vi "Create Tree.vi"(8 "Error In":errorcluster, 10 "Eulogy Bookmarks":T1[](array[typedef]), 11 "TreeControl In":refnum<vi>) -> (0 "Error Out":errorcluster, 3 "TreeControl Out":refnum<vi>)   [LabVIEW 2017, in "Bookmark Manager.lvlib"]
uses:
  Bookmark Manager.lvlib
  Controls/VI Bookmark.ctl
  Controls/VI Information.ctl
  Controls/Application Information.ctl
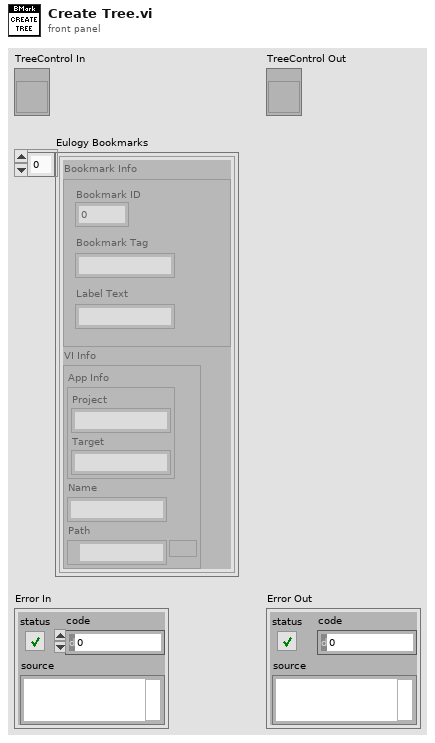
[diagram p1: front panel]
types:
  T1 = typedef "Bookmark Manager.lvlib/VI Bookmark.ctl" = cluster{"Bookmark Info":cluster{"Bookmark ID":u32, "Bookmark Tag":string, "Label Text":string}, "VI Info":T2}
  T2 = typedef "Bookmark Manager.lvlib/VI Information.ctl" = cluster{"App Info":T3, "Name":string, "Path":path}
  T3 = typedef "Bookmark Manager.lvlib/Application Information.ctl" = cluster{"Project":string, "Target":string}
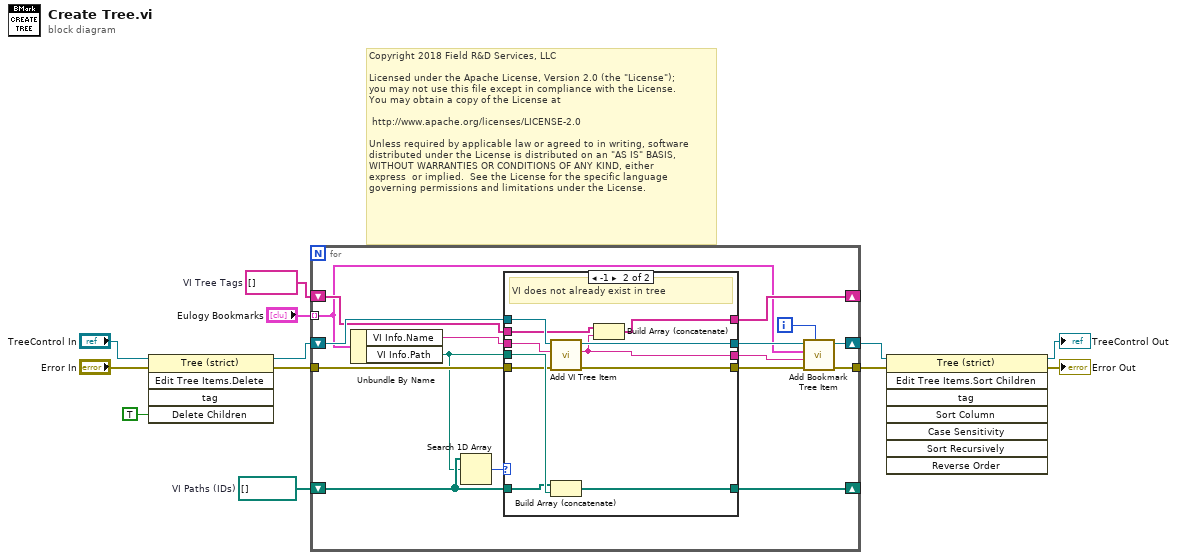
[diagram p0: block diagram]
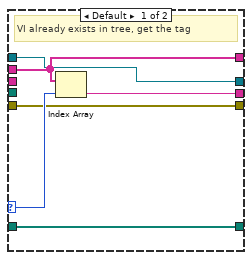
[diagram p2: hidden frame]
diagram:
  w1 = string[] []  # VI Tree Tags
  w2 = path[] []  # VI Paths (IDs)
  # "Copyright 2018 Field R&D Services, LLC\n\nLicensed under the Apache License, Version 2.0 (the \"License\");\nyou may not use this file except in compliance with the License.\nYou may obtain a copy of the License at\n\n\thttp://www.apache.org/licenses/LICENSE-2.0\n\nUnless required by applicable law or agreed to in writing, software\ndistributed under the License is distributed on an \"AS IS\" BASIS,\nWITHOUT WARRANTIES OR CONDITIONS OF ANY KIND, either \nexpress  or implied.  See the License for the specific language \ngoverning permissions and limitations under the License."
  n1 = invoke class="Tree (strict)" method="Edit Tree Items.Delete"(reference="TreeControl In", error in="Error In", "Delete Children"=TRUE ("Delete Children?")) -> (reference out=w7:refnum<vi>, error out=w9:errorcluster)  [unwired: 2 in, 3 out]
  n2 = for {
    shift-right: [w17] -> w8
    shift-left: w7 -> [w27]
    tunnel: w9 -> [w28]
    tunnel: [w16] -> w11
    tunnel: "Eulogy Bookmarks" -> [w13] mode=indexing
    shift-right: [w23] -> _
    shift-left: w2 -> [w24]
    shift-right: [w22] -> _
    shift-left: w1 -> [w21]
    i -> [w18]
    n3 = Unbundle By Name(w13) -> ("VI Info.Name"=w14:string, "VI Info.Path"=w15:path)
    n4 = Search 1D Array(1D array=w24, element=w15) -> (index of element=w25:i32)  [unwired: 1 in]
    n5 = case shown="-1" w25 {
      selector: w25 -> [w33 _]
      tunnel: w28 -> [w30 w35]
      tunnel: w27 -> [w34 w45]
      tunnel: [w34 w44] -> w26
      tunnel: w14 -> [_ w36]
      tunnel: w15 -> [_ w43]
      tunnel: w24 -> [w29 w42]
      tunnel: [w29 w41] -> w23
      tunnel: [w31 w40] -> w20
      tunnel: [w32 w39] -> w22
      tunnel: w21 -> [w32 w38]
      tunnel: [w30 w37] -> w19
      frame Default {
        # "VI already exists in tree, get the tag"
        n6 = Index Array(array=w32, index=w33) -> (element=w31:string)
      }
      frame -1 {
        # "VI does not already exist in tree"
        n7 = call "Add VI Tree Item.vi"("Error In"=w35, "VI Name"=w36, "TreeControl In"=w45) -> ("Error Out"=w37:errorcluster, "VI Tree Tag"=w40:string, "TreeControl Out"=w44:refnum<vi>)  [unwired: 6 in]
        n8 = Build Array (concatenate)(w42, w43) -> (w41:path[])
        n9 = Build Array (concatenate)(w38, w40) -> (w39:string[])
      }
    }
    n10 = call "Add Bookmark Tree Item.vi"("Index"=w18, "Error In"=w19, "Parent Tag"=w20, "VI Bookmark"=w13, "TreeControl In"=w26) -> ("Error Out"=w16:errorcluster, "TreeControl Out"=w17:refnum<vi>)  [unwired: 5 in]
  }
  n11 = invoke class="Tree (strict)" method="Edit Tree Items.Sort Children"(reference=w8, error in=w11) -> (reference out=→"TreeControl Out":refnum<vi>, error out=→"Error Out":errorcluster)  [unwired: 6 in, 6 out]
